vi "Test Vector XControl.vi"() -> ()   [LabVIEW 2012]
uses:
  Vector Function Generator.xctl
panel:
  in  "Go":bool
  in  "Vect XControl":waveform(cdb)(xcontrol)
  in  "Exit":bool
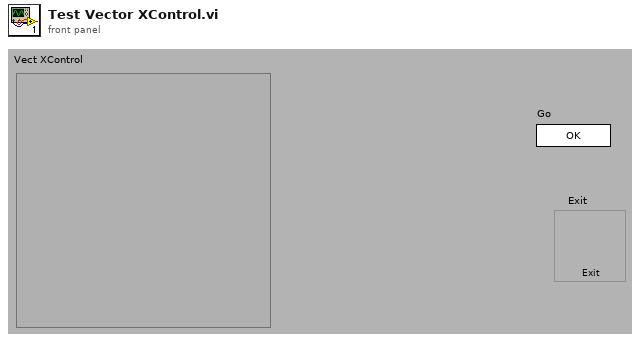
[diagram p1: front panel]
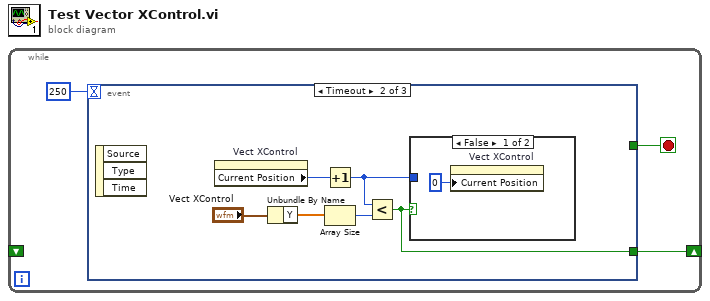
[diagram p0: block diagram]
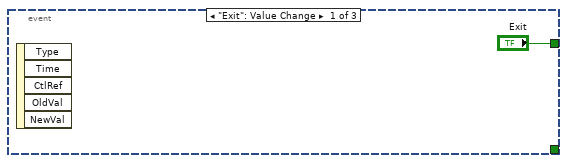
[diagram p2: hidden frame]
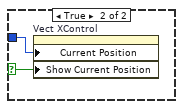
[diagram p3: hidden frame]
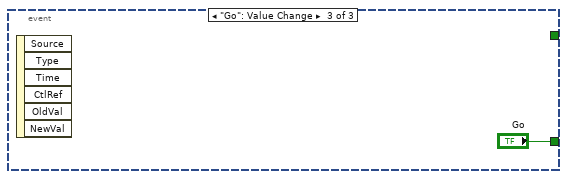
[diagram p4: hidden frame]
diagram:
  n1 = while {
    shift-right: [w2] -> _
    shift-left: _ -> [_]
    stop <- w3 stop-if-true
    n2 = event shown="[1] Timeout" {
      selector: _ -> [_ _ _]
      dyn-events: _ -> [_ _ _]
      timeout: 250 -> [_ _ _]
      tunnel: ["Exit" _ _] -> w3
      tunnel: [_ w5 "Go"] -> w2
      event "Exit": Value Change {
        n3 = event-data() -> ()  [unwired: 6 out]
      }
      event Timeout {
        n4 = event-data() -> ()  [unwired: 4 out]
        n5 = property on="Vect XControl" class="Vector Function Generator (stri"() -> ("Current Position"=w10:i32)  [unwired: 2 in, 2 out]
        n6 = Unbundle By Name("Vect XControl") -> ("Y"=w8:cdb[])
        n7 = Increment(x=w10) -> (x+1=w6:i32)
        n8 = Array Size(array=w8) -> (size(s)=w7:i32)
        n9 = Less?(x=w6, y=w7) -> (x < y?=w5:bool)
        n10 = case shown="False" w5 {
          selector: w5 -> [_ w13]
          tunnel: w6 -> [_ w12]
          frame False {
            n11 = property on="Vect XControl" class="Vector Function Generator (stri"("Current Position"=0) -> ()  [unwired: 2 in, 2 out]
          }
          frame True {
            n12 = property on="Vect XControl" class="Vector Function Generator (stri"("Current Position"=w12, "Show Current Position"=w13) -> ()  [unwired: 2 in, 2 out]
          }
        }
      }
      event "Go": Value Change {
        n13 = event-data() -> ()  [unwired: 7 out]
      }
    }
  }
